vi "Encode bytes.vi"(7 "Field Number":i32, 10 "bytes":u8[](array[numeric]) format="%.0x", 11 "Buffer in":u8[](array[numeric]) format="%.0x") -> (3 "Buffer":u8[](array[numeric]) format="%.0x")   [LabVIEW 2020, in "LV-Proto.lvlib"]
uses:
  LV-Proto.lvlib
  Wire Type.ctl
  Wire Encode Varint I32.vi
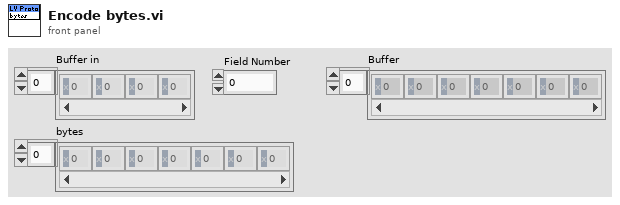
[diagram p1: front panel]
types:
  T1 = typedef "LV-Proto.lvlib/Wire Type.ctl" = enum8{"VARINT", "I64", "LEN", "SGROUP (Deprecated)", "EGROUP (Deprecated)", "I32"}
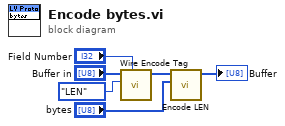
[diagram p0: block diagram]
diagram:
  n1 = call "Wire Encode Tag.vi"("Field Number"="Field Number", "Wire Type"=Wire_Type."LEN", "Buffer in"="Buffer in") -> ("Buffer"=w3:u8[])  [unwired: 8 in]
  n2 = call "Encode LEN.vi"("Data"="bytes", "Buffer in"=w3) -> ("Buffer"=→"Buffer":u8[])  [unwired: 9 in]
